vi "GetText.vi"(8 "error in":errorcluster, 11 "Simple Sequencer TBM editor node in":refnum<class "Simple Sequencer TBM editor node.lvclass">) -> (0 "error out":errorcluster, 1 "additional text":string, 2 "text":string, 3 "Simple Sequencer TBM editor node out":refnum<class "Simple Sequencer TBM editor node.lvclass">, 4 "glyph":string)   [LabVIEW 2015, in "Simple Sequencer TBM editor node.lvclass"]
uses:
  Simple Sequencer TBM editor node.lvclass
  module/configuration/Simple Sequencer TBM configuration.lvclass
  module/configuration/Simple Sequencer TBM configuration.lvclass/Simple Sequencer TBM configuration.ctl
  module/configuration/Write sequencer name.vi
  module/configuration/Read sequencer name.vi
  <vilib>/NI/DCAF/Tag Editor Core/Configuration Editor/Classes/Module editor node/Read Module Configuration.vi
  <vilib>/NI/DCAF/Tag Editor Core/Configuration Editor/Classes/Module editor node/Write Module Configuration.vi
  <vilib>/NI/Tag Bus Module Framework/module configuration/TBM module configuration.lvclass
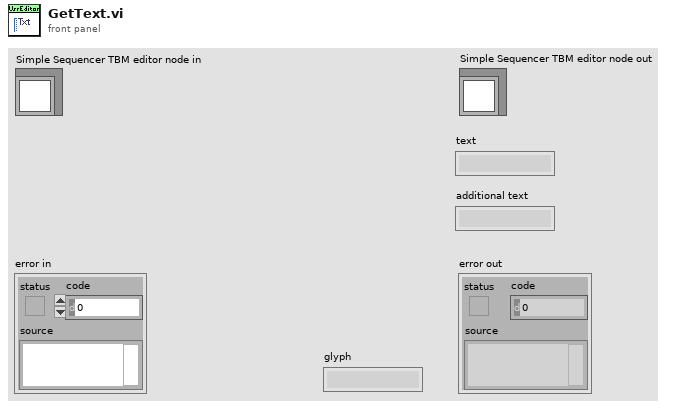
[diagram p1: front panel]
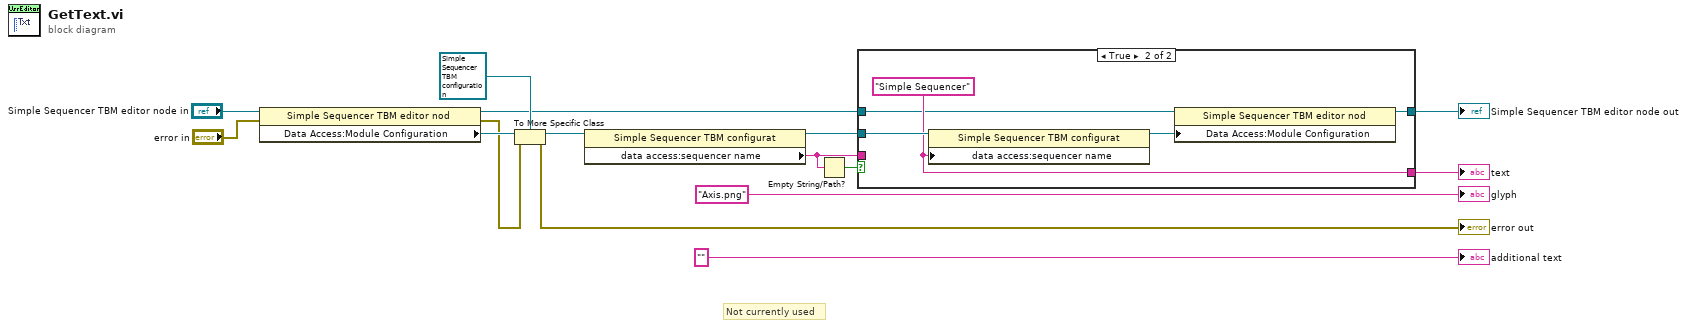
[diagram p0: block diagram]
diagram:
  # "Not currently used"
  n1 = property class="Simple Sequencer TBM editor nod"(reference="Simple Sequencer TBM editor node in", error in="error in") -> (reference out=w4:refnum<class "Simple Sequencer TBM editor node.lvclass">, error out=w10:errorcluster, "Data Access:Module Configuration"=w11:refnum<class "TBM module configuration.lvclass">)
  n2 = To More Specific Class(target class=refnum<class "Simple Sequencer TBM configuration.lvclass"> refnum ("Simple Sequencer TBM configuration"), reference=w11, error in=w10) -> (specific class reference=w8:refnum<class "Simple Sequencer TBM configuration.lvclass">, error out=→"error out":errorcluster)
  n3 = property class="Simple Sequencer TBM configurat"(reference=w8) -> (reference out=w5:refnum<class "Simple Sequencer TBM configuration.lvclass">, "data access:sequencer name"=w6:string)  [unwired: 1 in, 1 out]
  n4 = Empty String/Path?(string/path=w6) -> (empty?=w7:bool)
  n5 = case shown="True" w7 {
    tunnel: w6 -> [w17 _]
    tunnel: w5 -> [_ w22]
    tunnel: w4 -> [w16 w20]
    tunnel: [w17 w21] -> w3
    tunnel: [w16 w18] -> w2
    frame False {
    }
    frame True {
      w21 = "Simple Sequencer"
      n6 = property class="Simple Sequencer TBM configurat"(reference=w22, "data access:sequencer name"=w21) -> (reference out=w19:refnum<class "Simple Sequencer TBM configuration.lvclass">)  [unwired: 1 in, 1 out]
      n7 = property class="Simple Sequencer TBM editor nod"(reference=w20, "Data Access:Module Configuration"=w19) -> (reference out=w18:refnum<class "Simple Sequencer TBM editor node.lvclass">)  [unwired: 1 in, 1 out]
    }
  }
  "Simple Sequencer TBM editor node out" <- w2
  "text" <- w3
  "additional text" <- "" ("additional text")
  "glyph" <- "Axis.png" ("glyph")
